vi "Complementary Angle (array).vi"(7 "angle units":T1 items=["radian in, radian out", "radian in, degree out", "degree in, degree out", "degree in, radian out"], 11 "Angle":dbl[](array[numeric])) -> (0 "error":i32, 3 "Complementary Angle":dbl[](array[numeric]))   [LabVIEW 2020, in "NI_AAL_Angle.lvlib"]
doc: "Calculates the complementary angle of the input angle.\n\nWire data to any of the angle inputs to determine the polymorphic instance to use or manually select the instance."
uses:
  <vilib>/Analysis/NI_AAL_Angle.lvlib
  <vilib>/Analysis/coordinate.llb/Angle Units.ctl
  <vilib>/Analysis/coordinate.llb/Angle Range (Degree).ctl
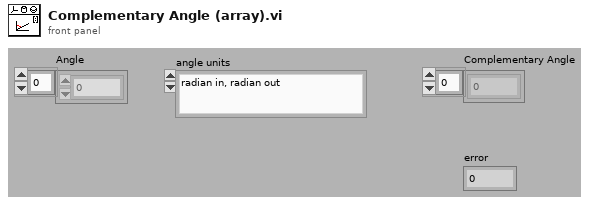
[diagram p1: front panel]
types:
  T1 = typedef "NI_AAL_Angle.lvlib/Angle Units.ctl" = i32
  T2 = typedef "NI_AAL_Angle.lvlib/Angle Range (Degree).ctl" = u16
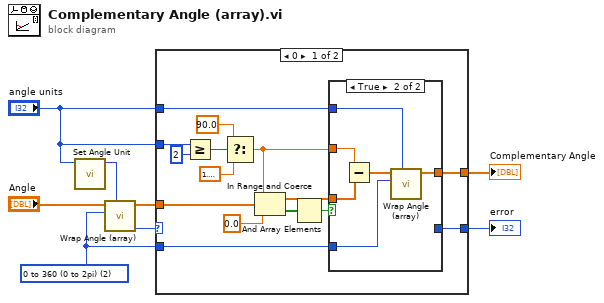
[diagram p0: block diagram]
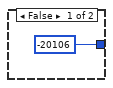
[diagram p2: hidden frame]
diagram:
  w4 = T2 2 items=["none", "-180 to 180 (-pi to pi)", "0 to 360 (0 to 2pi)"] ("angle range")
  n1 = call <vilib>:"Set Angle Unit.vi"("angle units in"="angle units") -> ("angle units out"=w8:T1)  [unwired: 10 in]
  n2 = call <vilib>:"Wrap Angle (array).vi"("angle units"=w8, "angle range"=w4, "Angle In"="Angle") -> ("error"=w6:i32, "Angle Out"=w3:dbl[])  [unwired: 7 in]
  n3 = case shown="0" w6 {
    selector: w6 -> [_ w31]
    tunnel: w3 -> [w23 _]
    tunnel: "angle units" -> [w22 _]
    tunnel: [w14 _] -> w2
    tunnel: [w13 w31] -> w1
    tunnel: "angle units" -> [w12 _]
    tunnel: w4 -> [w11 _]
    frame 0 {
      n4 = Greater Or Equal?(x=w22, y=2) -> (x >= y?=w19:bool)
      n5 = Select(t=90.0, s=w19, f=1.5707963267948966) -> (s? t:f=w15:dbl)
      n6 = In Range and Coerce(upper limit=w15, x=w23, lower limit=0.0 ("upper limit")) -> (coerced(x)=w16:dbl[], In Range?=w9:bool[])
      n7 = And Array Elements(Boolean array=w9) -> (logical AND=w10:bool)
      n8 = case shown="True" w10 {
        tunnel: w16 -> [_ w30]
        tunnel: w15 -> [_ w29]
        tunnel: [_ w27] -> w14
        tunnel: [-20106 _] -> w13
        tunnel: w12 -> [_ w26]
        tunnel: w11 -> [_ w25]
        frame False {
        }
        frame True {
          n9 = Subtract(x=w29, y=w30) -> (x-y=w28:dbl[])
          n10 = call <vilib>:"Wrap Angle (array).vi"("angle units"=w26, "angle range"=w25, "Angle In"=w28) -> ("Angle Out"=w27:dbl[])  [unwired: 7 in, 1 out]
        }
      }
    }
    frame 1, Default {
    }
  }
  "Complementary Angle" <- w2
  "error" <- w1
